vi "Timing_WireDelay.vi"(7 "milliseconds to wait":u32, 10 "Error In":errorcluster) -> (2 "Error Out":errorcluster, 5 "millisecond timer value":u32)   [LabVIEW 2017]
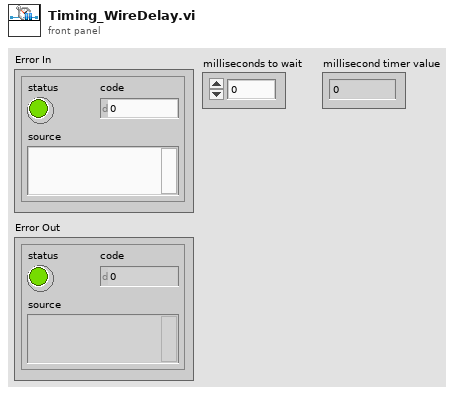
[diagram p1: front panel]
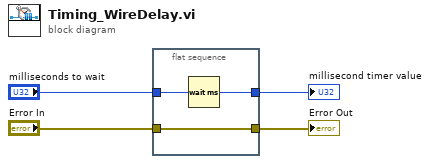
[diagram p0: block diagram]
diagram:
  n1 = flat-sequence {
    tunnel: "milliseconds to wait" -> [w7]
    tunnel: [w6] -> w3
    tunnel: [w5] -> w1
    tunnel: "Error In" -> [w5]
    frame #0 {
      n2 = Wait (ms)(milliseconds to wait=w7) -> (millisecond timer value=w6:u32)
    }
  }
  "Error Out" <- w1
  "millisecond timer value" <- w3
